vi "Stop Core.vi"(10 "final error code":i32 caption="最终错误代码", 11 "DAM0200-Relay in":refnum<class "DAM0200-Relay.lvclass"> caption="操作者输入") -> (3 "DAM0200-Relay out":refnum<class "DAM0200-Relay.lvclass"> caption="操作者输出")   [LabVIEW 2016, in "DAM0200-Relay.lvlib" / "DAM0200-Relay.lvclass"]
doc: "(<B>Filename</B>: Actor Framework.lvlib:Actor.lvclass:Stop Core.vi)\n\nDefines what the actor does before it stops. Use the <B>final error code</B> input to determine whether the actor shut down in response to an error.\n\nBy default, this method does nothing.子孙类重写该方法，定义出错时的操作，例如，关闭操作者核心方法初始的进程。"
uses:
  DAM0200-Relay.lvclass
  <vilib>/ActorFramework/Actor/Actor.lvclass
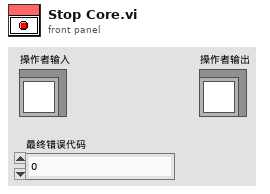
[diagram p1: front panel]
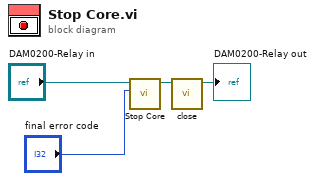
[diagram p0: block diagram]
diagram:
  n1 = call-parent "Stop Core.vi"("final error code"="final error code", "Actor in"="DAM0200-Relay in") -> ("Actor out"=w2:refnum<class "DAM0200-Relay.lvclass">)  [unwired: 9 in]
  n2 = call "close.vi"("DAM0200-Relay 输入"=w2) -> ("DAM0200-Relay 输出"=→"DAM0200-Relay out":refnum<class "DAM0200-Relay.lvclass">)  [unwired: 9 in, 1 out]
